vi "PSU_Keysight_34951A_SoftFP.vi"(0 "reference in":refnum<class "PSU_Keysight_34951A.lvclass">, 2 "Floating":bool, 5 "error in (no error)":errorcluster) -> (14 "reference out":refnum<class "PSU_Keysight_34951A.lvclass">, 19 "error out":errorcluster)   [LabVIEW 2022 SP3, in "PSU_Keysight_34951A.lvlib" / "PSU_Keysight_34951A.lvclass"]
uses:
  PSU_Keysight_34951A.lvclass
  Components/ViPER.lvlibp/ViPER.lvclass
  C:/Projects/Medulla/ViPER/Examples/Flux_Capacitor_Tester/Components/ViPER.lvlibp/ViPER.lvclass
panel:
  in  "C 4":T1 {"Current (A)" min=-0.02 max=0.02 step=0.001; "Voltage (V)" min=-16.0 max=16.0 step=0.01}
  in  "C 3":T1 {"Current (A)" min=-0.02 max=0.02 step=0.001; "Voltage (V)" min=-16.0 max=16.0 step=0.01}
  in  "C 2":T1 {"Current (A)" min=-0.02 max=0.02 step=0.001; "Voltage (V)" min=-16.0 max=16.0 step=0.01}
  in  "C1":T1 {"Current (A)" min=-0.02 max=0.02 step=0.001; "Voltage (V)" min=-16.0 max=16.0 step=0.01}
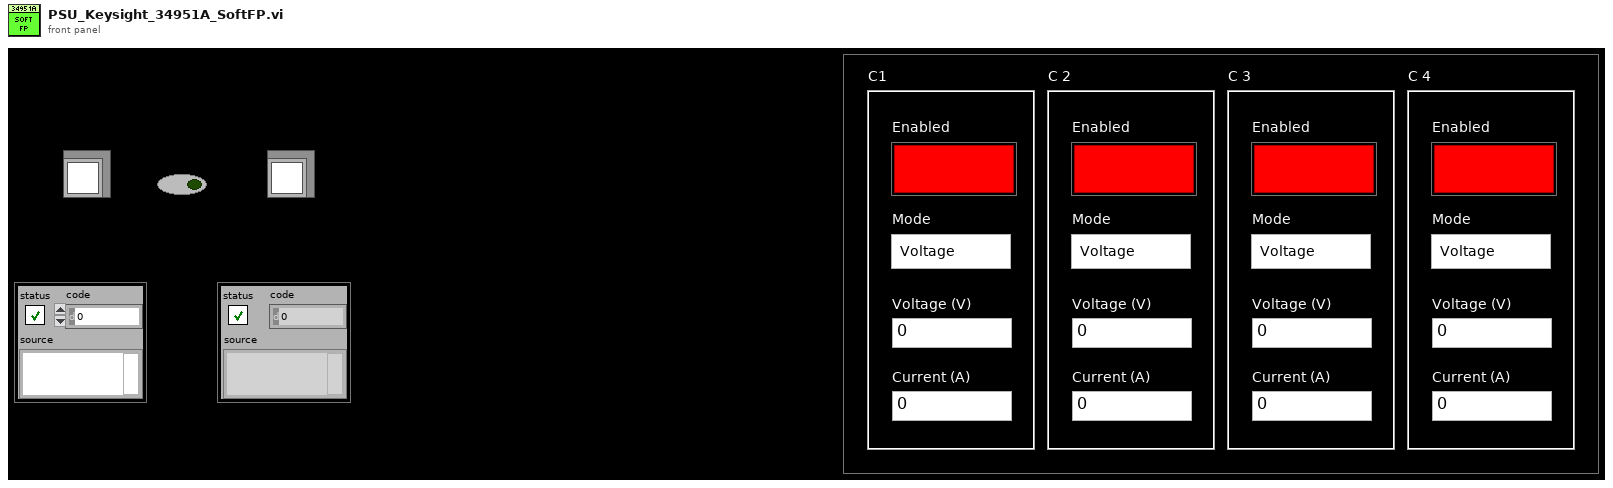
[diagram p1: front panel]
types:
  T1 = cluster{"Enabled":bool, "Mode":enum16{"Voltage", "Current"}, "Voltage (V)":dbl, "Current (A)":dbl}
  T2 = enum32{"Invalid", "Standard", "Closed", "Hidden", "Minimized", "Maximized"}
  T3 = typedef "PSU_Keysight_34951A.lvlib/PSU_Keysight_34951A.lvclass/ObjectAttributes.ctl" = cluster{"Config":T4, "VISA res":refnum<visa-resource-name>, "Enabled":bool[], "V":dbl[], "I":dbl[], "Source Type":enum16{"Voltage", "Current"}[]}
  T4 = typedef "PSU_Keysight_34951A.lvlib/PSU_Keysight_34951A.lvclass/Config.ctl" = cluster{"VISA":refnum<visa-resource-name>, "Slot":i32}
  T5 = cluster{"Enabled":bool, "Mode":bool, "Voltage (V)":bool, "Current (A)":bool}
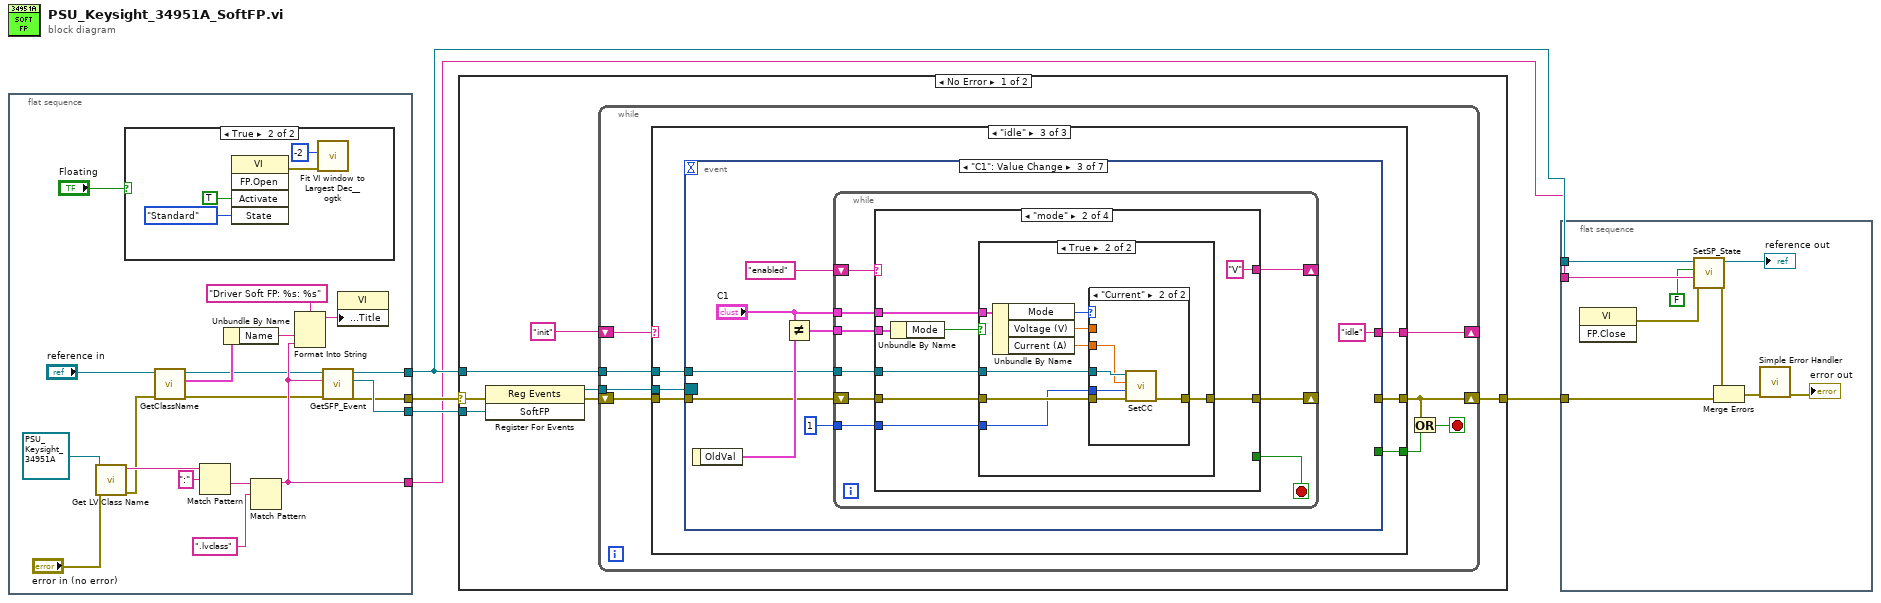
[diagram p0: block diagram]
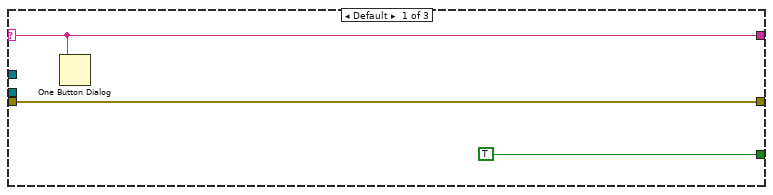
[diagram p3: hidden frame]
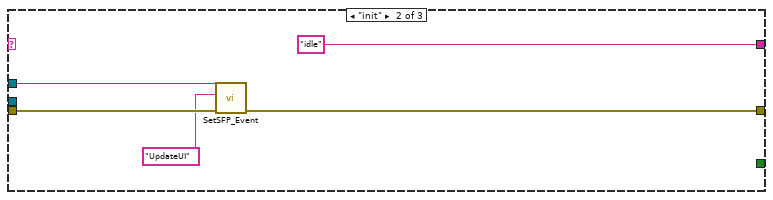
[diagram p4: hidden frame]
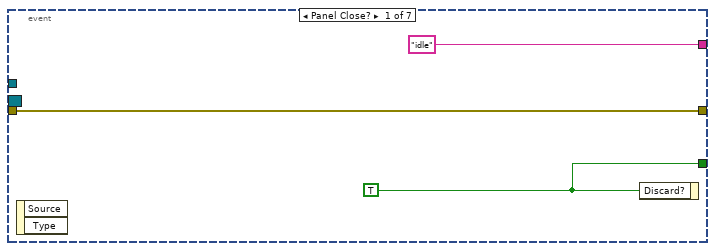
[diagram p5: hidden frame]
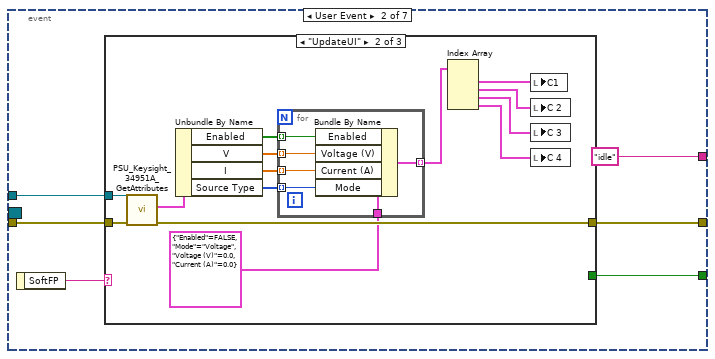
[diagram p6: hidden frame]
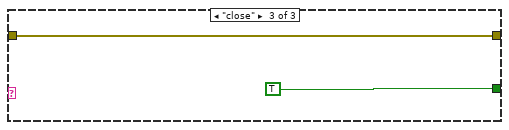
[diagram p8: hidden frame]
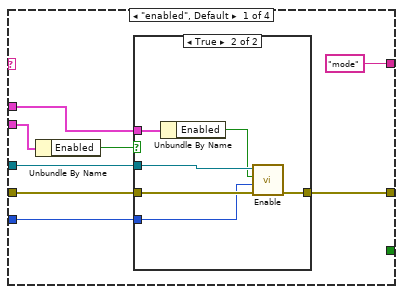
[diagram p9: hidden frame]
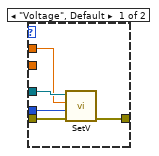
[diagram p12: hidden frame]
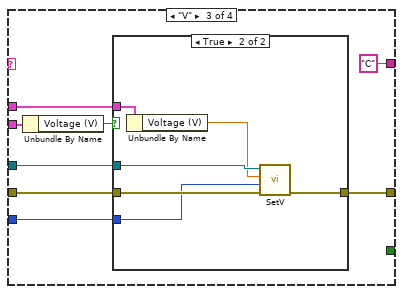
[diagram p13: hidden frame]
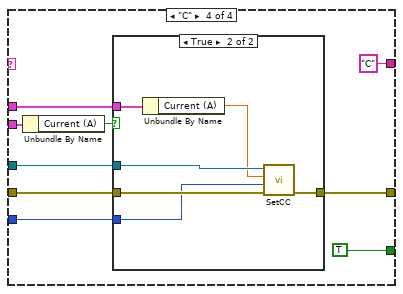
[diagram p15: hidden frame]
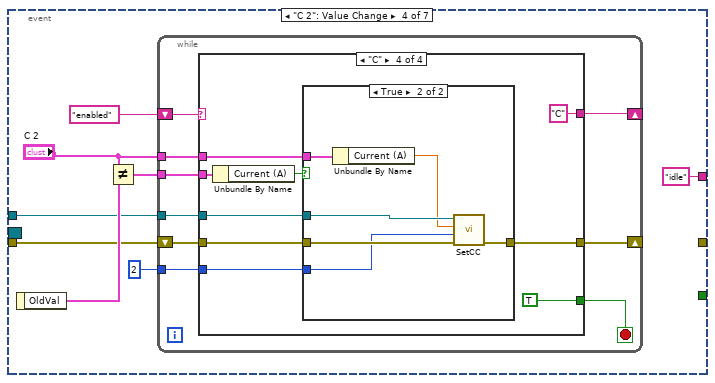
[diagram p17: hidden frame]
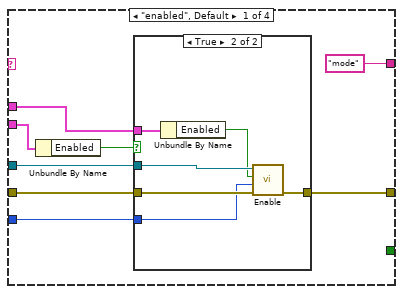
[diagram p18: hidden frame]
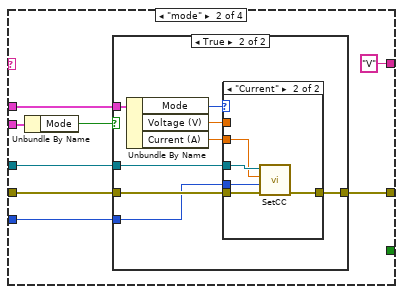
[diagram p20: hidden frame]
diagram:
  n1 = flat-sequence {
    tunnel: [w21] -> w5
    tunnel: [w20] -> w2
    tunnel: [w24] -> w3
    tunnel: [w12] -> w1
    frame #0 {
      n2 = call <vilib>:"Get LV Class Name.vi"("error in (no error)"="error in (no error)", "object"=refnum<class "PSU_Keysight_34951A.lvclass"> refnum ("reference")) -> ("error out"=w11:errorcluster, "class name"=w17:string)  [unwired: 8 in]
      n3 = case shown="True" "Floating" {
        frame False {
        }
        frame True {
          n4 = invoke class="VI" method="FP.Open"("Activate"=TRUE ("Activate?"), "State"=T2."Standard") -> (error out=w25:errorcluster)  [unwired: 3 in, 4 out]
          n5 = call <userlib>:"Fit VI window to Largest Dec__ogtk.vi"("error in (no error)"=w25, "border spacing (2 px)"=-2) -> ()  [unwired: 4 in, 2 out]
        }
      }
      n6 = call "GetClassName.vi"("error in (no error)"=w11, "reference in"="reference in") -> ("error out"=w10:errorcluster, "Details"=w9:cluster{"Name":string, "Class":string}, "reference out"=w7:refnum<class "PSU_Keysight_34951A.lvclass">)  [unwired: 7 in]
      n7 = Match Pattern(string=w17, regular expression=":") -> (after substring=w15:string)  [unwired: 1 in, 3 out]
      n8 = Unbundle By Name(w9) -> ("Name"=w19:string)
      n9 = Match Pattern(string=w15, regular expression=".lvclass") -> (before substring=w12:string)  [unwired: 1 in, 3 out]
      n10 = Format Into String(format string="Driver Soft FP: %s: %s", w19, w12) -> (resulting string=w23:string)  [unwired: 2 in, 1 out]
      n11 = call-dynamic "GetSFP_Event.vi"("error in (no error)"=w10, "Ancestor"=w12, "reference in"=w7) -> ("error out"=w21:errorcluster, "SoftFP"=w24:refnum<user-event>, "reference out"=w20:refnum<class "PSU_Keysight_34951A.lvclass">)  [unwired: 6 in]
      n12 = property class="VI"("Front Panel.Title"=w23) -> ()  [unwired: 2 in, 2 out]
    }
  }
  n13 = case shown="No Error" w5 {
    selector: w5 -> [w33 w452]
    tunnel: [w29 w452] -> w4
    tunnel: w2 -> [w30 _]
    tunnel: w3 -> [w35 _]
    frame No Error {
      n14 = register-events(error in=w33, w35) -> (reference out=w34:refnum<event-registration>, error out=w32:errorcluster)  [unwired: 1 in]
      n15 = while {
        shift-right: [w40] -> w29
        shift-left: w32 -> [w43]
        tunnel: w34 -> [w42]
        tunnel: w30 -> [w41]
        shift-right: [w36] -> _
        shift-left: "init" -> [w37]
        stop <- w39 stop-if-true
        n16 = case shown="\"idle\"" w37 {
          selector: w37 -> [w44 _ _]
          tunnel: w43 -> [w45 w49 w57]
          tunnel: w42 -> [_ _ w56]
          tunnel: w41 -> [_ w48 w55]
          tunnel: [w45 w50 w54] -> w40
          tunnel: [TRUE ("Discard?") _ w53] -> w38
          tunnel: [w44 "idle" w52] -> w36
          frame Default {
            n17 = One Button Dialog(message=w44) -> ()  [unwired: 1 in, 1 out]
          }
          frame "init" {
            n18 = call-dynamic "SetSFP_Event.vi"("error in (no error)"=w49, "msg"="UpdateUI" ("Ancestor"), "reference in"=w48) -> ("error out"=w50:errorcluster)  [unwired: 7 in, 1 out]
          }
          frame "idle" {
            n19 = event shown="[2] \"C1\": Value Change" {
              selector: w56 -> [_ _ _ _ _ _ _]
              dyn-events: _ -> [_ _ _ _ _ _ _]
              timeout: _ -> [_ _ _ _ _ _ _]
              tunnel: w57 -> [w60 w66 w91 w182 w272 w362 w451]
              tunnel: [w60 w64 _ _ _ _ w451] -> w54
              tunnel: [w59 w63 _ _ _ _ _] -> w53
              tunnel: w55 -> [_ w61 w90 w181 w271 w361 _]
              tunnel: ["idle" "idle" "idle" "idle" "idle" "idle" "idle"] -> w52
              event Panel Close? {
                w59 = TRUE ("Discard?")
                n20 = event-data() -> ()  [unwired: 1 in, 2 out]
                n21 = event-data("Discard?"=w59) -> ()  [unwired: 1 in, 1 out]
              }
              event User Event {
                n22 = event-data() -> ("SoftFP"=w65:string)  [unwired: 1 in]
                n23 = case shown="\"UpdateUI\"" w65 {
                  tunnel: w66 -> [w67 w81 w89]
                  tunnel: [w67 w79 w89] -> w64
                  tunnel: [_ _ TRUE ("Discard?")] -> w63
                  tunnel: w61 -> [_ w80 _]
                  frame Default {
                  }
                  frame "UpdateUI" {
                    n24 = call "PSU_Keysight_34951A_GetAttributes.vi"("error in (no error)"=w81, "reference in"=w80) -> ("error out"=w79:errorcluster, "Data"=w78:T3)  [unwired: 6 in, 2 out]
                    n25 = Unbundle By Name(w78) -> ("Enabled"=w77:bool[], "V"=w76:dbl[], "I"=w75:dbl[], "Source Type"=w74:enum16{"Voltage", "Current"}[])
                    n26 = for {
                      tunnel: w77 -> [w86] mode=indexing
                      tunnel: w76 -> [w85] mode=indexing
                      tunnel: w75 -> [w84] mode=indexing
                      tunnel: w74 -> [w83] mode=indexing
                      tunnel: T1 {"Enabled"=FALSE, "Mode"=enum."Voltage", "Voltage (V)"=0.0, "Current (A)"=0.0} ("C1") -> [w87]
                      tunnel: [w82] -> w72 mode=indexing
                      n27 = Bundle By Name(cluster=w87, "Enabled"=w86, "Voltage (V)"=w85, "Current (A)"=w84, "Mode"=w83) -> (w82:T1)
                    }
                    n28 = Index Array(array=w72) -> (element #1=w71:T1, element #2=w70:T1, element #3=w69:T1, element #4=w68:T1)  [unwired: 4 in]
                    n29 = local write "C1"(w71) -> ()
                    n30 = local write "C 2"(w70) -> ()
                    n31 = local write "C 3"(w69) -> ()
                    n32 = local write "C 4"(w68) -> ()
                  }
                  frame "close" {
                  }
                }
              }
              event "C1": Value Change {
                n33 = event-data() -> ("OldVal"=w97:T1)  [unwired: 1 in]
                n34 = Not Equal?(x="C1", y=w97) -> (x != y?=w95:T5)
                n35 = while {
                  tunnel: w95 -> [w105]
                  shift-right: [w98] -> _
                  shift-left: "enabled" -> [w106]
                  tunnel: "C1" -> [w104]
                  tunnel: 1 -> [w103]
                  shift-right: [w100] -> _
                  shift-left: w91 -> [w102]
                  tunnel: w90 -> [w101]
                  stop <- w99 stop-if-true
                  n36 = case shown="\"mode\"" w106 {
                    tunnel: w105 -> [w114 w129 w156 w172]
                    tunnel: w104 -> [w112 w127 w154 w170]
                    tunnel: w103 -> [w109 w124 w151 w167]
                    tunnel: w102 -> [w111 w126 w153 w169]
                    tunnel: w101 -> [w110 w125 w152 w168]
                    tunnel: [w108 w123 w150 w166] -> w100
                    tunnel: [_ _ _ TRUE] -> w99
                    tunnel: ["mode" "V" "C" "C"] -> w98
                    frame "enabled", Default {
                      n37 = Unbundle By Name(w114) -> ("Enabled"=w113:bool)
                      n38 = case shown="True" w113 {
                        tunnel: w112 -> [_ w121]
                        tunnel: w111 -> [w115 w119]
                        tunnel: w110 -> [_ w120]
                        tunnel: w109 -> [_ w117]
                        tunnel: [w115 w116] -> w108
                        frame False {
                        }
                        frame True {
                          n39 = Unbundle By Name(w121) -> ("Enabled"=w118:bool)
                          n40 = call-dynamic "Enable.vi"("error in (no error)"=w119, "Chan"=w117, "Enable"=w118, "reference in"=w120) -> ("error out"=w116:errorcluster)  [unwired: 6 in, 1 out]
                        }
                      }
                    }
                    frame "mode" {
                      n41 = Unbundle By Name(w129) -> ("Mode"=w128:bool)
                      n42 = case shown="True" w128 {
                        tunnel: w127 -> [_ w138]
                        tunnel: w126 -> [w130 w136]
                        tunnel: w125 -> [_ w137]
                        tunnel: w124 -> [_ w135]
                        tunnel: [w130 w134] -> w123
                        frame False {
                        }
                        frame True {
                          n43 = Unbundle By Name(w138) -> ("Mode"=w133:enum16{"Voltage", "Current"}, "Voltage (V)"=w132:dbl, "Current (A)"=w131:dbl)
                          n44 = case shown="\"Current\"" w133 {
                            tunnel: w137 -> [w141 w146]
                            tunnel: w136 -> [w143 w148]
                            tunnel: w135 -> [w140 w144]
                            tunnel: [w142 w147] -> w134
                            tunnel: w132 -> [w139 _]
                            tunnel: w131 -> [_ w145]
                            frame "Voltage", Default {
                              n45 = call-dynamic "SetV.vi"("error in (no error)"=w143, "Chan"=w140, "V"=w139, "reference in"=w141) -> ("error out"=w142:errorcluster)  [unwired: 6 in, 1 out]
                            }
                            frame "Current" {
                              n46 = call-dynamic "SetCC.vi"("error in (no error)"=w148, "Chan"=w144, "CC"=w145, "reference in"=w146) -> ("error out"=w147:errorcluster)  [unwired: 6 in, 1 out]
                            }
                          }
                        }
                      }
                    }
                    frame "V" {
                      n47 = Unbundle By Name(w156) -> ("Voltage (V)"=w155:bool)
                      n48 = case shown="True" w155 {
                        tunnel: w154 -> [_ w163]
                        tunnel: w153 -> [w157 w161]
                        tunnel: w152 -> [_ w162]
                        tunnel: w151 -> [_ w160]
                        tunnel: [w157 w159] -> w150
                        frame False {
                        }
                        frame True {
                          n49 = Unbundle By Name(w163) -> ("Voltage (V)"=w158:dbl)
                          n50 = call-dynamic "SetV.vi"("error in (no error)"=w161, "Chan"=w160, "V"=w158, "reference in"=w162) -> ("error out"=w159:errorcluster)  [unwired: 6 in, 1 out]
                        }
                      }
                    }
                    frame "C" {
                      n51 = Unbundle By Name(w172) -> ("Current (A)"=w171:bool)
                      n52 = case shown="True" w171 {
                        tunnel: w170 -> [_ w179]
                        tunnel: w169 -> [w173 w178]
                        tunnel: w168 -> [_ w176]
                        tunnel: w167 -> [_ w174]
                        tunnel: [w173 w177] -> w166
                        frame False {
                        }
                        frame True {
                          n53 = Unbundle By Name(w179) -> ("Current (A)"=w175:dbl)
                          n54 = call-dynamic "SetCC.vi"("error in (no error)"=w178, "Chan"=w174, "CC"=w175, "reference in"=w176) -> ("error out"=w177:errorcluster)  [unwired: 6 in, 1 out]
                        }
                      }
                    }
                  }
                }
              }
              event "C 2": Value Change {
                n55 = event-data() -> ("OldVal"=w187:T1)  [unwired: 1 in]
                n56 = Not Equal?(x="C 2", y=w187) -> (x != y?=w185:T5)
                n57 = while {
                  tunnel: w185 -> [w195]
                  shift-right: [w188] -> _
                  shift-left: "enabled" -> [w196]
                  tunnel: "C 2" -> [w194]
                  tunnel: 2 -> [w193]
                  shift-right: [w190] -> _
                  shift-left: w182 -> [w192]
                  tunnel: w181 -> [w191]
                  stop <- w189 stop-if-true
                  n58 = case shown="\"C\"" w196 {
                    tunnel: w195 -> [w204 w219 w246 w262]
                    tunnel: w194 -> [w202 w217 w244 w260]
                    tunnel: w193 -> [w199 w214 w241 w257]
                    tunnel: w192 -> [w201 w216 w243 w259]
                    tunnel: w191 -> [w200 w215 w242 w258]
                    tunnel: [w198 w213 w240 w256] -> w190
                    tunnel: [_ _ _ TRUE] -> w189
                    tunnel: ["mode" "V" "C" "C"] -> w188
                    frame "enabled", Default {
                      n59 = Unbundle By Name(w204) -> ("Enabled"=w203:bool)
                      n60 = case shown="True" w203 {
                        tunnel: w202 -> [_ w211]
                        tunnel: w201 -> [w205 w209]
                        tunnel: w200 -> [_ w210]
                        tunnel: w199 -> [_ w207]
                        tunnel: [w205 w206] -> w198
                        frame False {
                        }
                        frame True {
                          n61 = Unbundle By Name(w211) -> ("Enabled"=w208:bool)
                          n62 = call-dynamic "Enable.vi"("error in (no error)"=w209, "Chan"=w207, "Enable"=w208, "reference in"=w210) -> ("error out"=w206:errorcluster)  [unwired: 6 in, 1 out]
                        }
                      }
                    }
                    frame "mode" {
                      n63 = Unbundle By Name(w219) -> ("Mode"=w218:bool)
                      n64 = case shown="True" w218 {
                        tunnel: w217 -> [_ w228]
                        tunnel: w216 -> [w220 w226]
                        tunnel: w215 -> [_ w227]
                        tunnel: w214 -> [_ w225]
                        tunnel: [w220 w224] -> w213
                        frame False {
                        }
                        frame True {
                          n65 = Unbundle By Name(w228) -> ("Mode"=w223:enum16{"Voltage", "Current"}, "Voltage (V)"=w222:dbl, "Current (A)"=w221:dbl)
                          n66 = case shown="\"Current\"" w223 {
                            tunnel: w227 -> [w231 w236]
                            tunnel: w226 -> [w233 w238]
                            tunnel: w225 -> [w230 w234]
                            tunnel: [w232 w237] -> w224
                            tunnel: w222 -> [w229 _]
                            tunnel: w221 -> [_ w235]
                            frame "Voltage", Default {
                              n67 = call-dynamic "SetV.vi"("error in (no error)"=w233, "Chan"=w230, "V"=w229, "reference in"=w231) -> ("error out"=w232:errorcluster)  [unwired: 6 in, 1 out]
                            }
                            frame "Current" {
                              n68 = call-dynamic "SetCC.vi"("error in (no error)"=w238, "Chan"=w234, "CC"=w235, "reference in"=w236) -> ("error out"=w237:errorcluster)  [unwired: 6 in, 1 out]
                            }
                          }
                        }
                      }
                    }
                    frame "V" {
                      n69 = Unbundle By Name(w246) -> ("Voltage (V)"=w245:bool)
                      n70 = case shown="True" w245 {
                        tunnel: w244 -> [_ w253]
                        tunnel: w243 -> [w247 w251]
                        tunnel: w242 -> [_ w252]
                        tunnel: w241 -> [_ w250]
                        tunnel: [w247 w249] -> w240
                        frame False {
                        }
                        frame True {
                          n71 = Unbundle By Name(w253) -> ("Voltage (V)"=w248:dbl)
                          n72 = call-dynamic "SetV.vi"("error in (no error)"=w251, "Chan"=w250, "V"=w248, "reference in"=w252) -> ("error out"=w249:errorcluster)  [unwired: 6 in, 1 out]
                        }
                      }
                    }
                    frame "C" {
                      n73 = Unbundle By Name(w262) -> ("Current (A)"=w261:bool)
                      n74 = case shown="True" w261 {
                        tunnel: w260 -> [_ w269]
                        tunnel: w259 -> [w263 w268]
                        tunnel: w258 -> [_ w266]
                        tunnel: w257 -> [_ w264]
                        tunnel: [w263 w267] -> w256
                        frame False {
                        }
                        frame True {
                          n75 = Unbundle By Name(w269) -> ("Current (A)"=w265:dbl)
                          n76 = call-dynamic "SetCC.vi"("error in (no error)"=w268, "Chan"=w264, "CC"=w265, "reference in"=w266) -> ("error out"=w267:errorcluster)  [unwired: 6 in, 1 out]
                        }
                      }
                    }
                  }
                }
              }
              event "C 3": Value Change {
                n77 = event-data() -> ("OldVal"=w277:T1)  [unwired: 1 in]
                n78 = Not Equal?(x="C 3", y=w277) -> (x != y?=w275:T5)
                n79 = while {
                  tunnel: w275 -> [w285]
                  shift-right: [w278] -> _
                  shift-left: "enabled" -> [w286]
                  tunnel: "C 3" -> [w284]
                  tunnel: 3 -> [w283]
                  shift-right: [w280] -> _
                  shift-left: w272 -> [w282]
                  tunnel: w271 -> [w281]
                  stop <- w279 stop-if-true
                  n80 = case shown="\"C\"" w286 {
                    tunnel: w285 -> [w294 w309 w336 w352]
                    tunnel: w284 -> [w292 w307 w334 w350]
                    tunnel: w283 -> [w289 w304 w331 w347]
                    tunnel: w282 -> [w291 w306 w333 w349]
                    tunnel: w281 -> [w290 w305 w332 w348]
                    tunnel: [w288 w303 w330 w346] -> w280
                    tunnel: [_ _ _ TRUE] -> w279
                    tunnel: ["mode" "V" "C" "C"] -> w278
                    frame "enabled", Default {
                      n81 = Unbundle By Name(w294) -> ("Enabled"=w293:bool)
                      n82 = case shown="True" w293 {
                        tunnel: w292 -> [_ w301]
                        tunnel: w291 -> [w295 w299]
                        tunnel: w290 -> [_ w300]
                        tunnel: w289 -> [_ w297]
                        tunnel: [w295 w296] -> w288
                        frame False {
                        }
                        frame True {
                          n83 = Unbundle By Name(w301) -> ("Enabled"=w298:bool)
                          n84 = call-dynamic "Enable.vi"("error in (no error)"=w299, "Chan"=w297, "Enable"=w298, "reference in"=w300) -> ("error out"=w296:errorcluster)  [unwired: 6 in, 1 out]
                        }
                      }
                    }
                    frame "mode" {
                      n85 = Unbundle By Name(w309) -> ("Mode"=w308:bool)
                      n86 = case shown="True" w308 {
                        tunnel: w307 -> [_ w318]
                        tunnel: w306 -> [w310 w316]
                        tunnel: w305 -> [_ w317]
                        tunnel: w304 -> [_ w315]
                        tunnel: [w310 w314] -> w303
                        frame False {
                        }
                        frame True {
                          n87 = Unbundle By Name(w318) -> ("Mode"=w313:enum16{"Voltage", "Current"}, "Voltage (V)"=w312:dbl, "Current (A)"=w311:dbl)
                          n88 = case shown="\"Current\"" w313 {
                            tunnel: w317 -> [w321 w326]
                            tunnel: w316 -> [w323 w328]
                            tunnel: w315 -> [w320 w324]
                            tunnel: [w322 w327] -> w314
                            tunnel: w312 -> [w319 _]
                            tunnel: w311 -> [_ w325]
                            frame "Voltage", Default {
                              n89 = call-dynamic "SetV.vi"("error in (no error)"=w323, "Chan"=w320, "V"=w319, "reference in"=w321) -> ("error out"=w322:errorcluster)  [unwired: 6 in, 1 out]
                            }
                            frame "Current" {
                              n90 = call-dynamic "SetCC.vi"("error in (no error)"=w328, "Chan"=w324, "CC"=w325, "reference in"=w326) -> ("error out"=w327:errorcluster)  [unwired: 6 in, 1 out]
                            }
                          }
                        }
                      }
                    }
                    frame "V" {
                      n91 = Unbundle By Name(w336) -> ("Voltage (V)"=w335:bool)
                      n92 = case shown="True" w335 {
                        tunnel: w334 -> [_ w343]
                        tunnel: w333 -> [w337 w341]
                        tunnel: w332 -> [_ w342]
                        tunnel: w331 -> [_ w340]
                        tunnel: [w337 w339] -> w330
                        frame False {
                        }
                        frame True {
                          n93 = Unbundle By Name(w343) -> ("Voltage (V)"=w338:dbl)
                          n94 = call-dynamic "SetV.vi"("error in (no error)"=w341, "Chan"=w340, "V"=w338, "reference in"=w342) -> ("error out"=w339:errorcluster)  [unwired: 6 in, 1 out]
                        }
                      }
                    }
                    frame "C" {
                      n95 = Unbundle By Name(w352) -> ("Current (A)"=w351:bool)
                      n96 = case shown="True" w351 {
                        tunnel: w350 -> [_ w359]
                        tunnel: w349 -> [w353 w358]
                        tunnel: w348 -> [_ w356]
                        tunnel: w347 -> [_ w354]
                        tunnel: [w353 w357] -> w346
                        frame False {
                        }
                        frame True {
                          n97 = Unbundle By Name(w359) -> ("Current (A)"=w355:dbl)
                          n98 = call-dynamic "SetCC.vi"("error in (no error)"=w358, "Chan"=w354, "CC"=w355, "reference in"=w356) -> ("error out"=w357:errorcluster)  [unwired: 6 in, 1 out]
                        }
                      }
                    }
                  }
                }
              }
              event "C 4": Value Change {
                n99 = event-data() -> ("OldVal"=w367:T1)  [unwired: 1 in]
                n100 = Not Equal?(x="C 4", y=w367) -> (x != y?=w365:T5)
                n101 = while {
                  tunnel: w365 -> [w375]
                  shift-right: [w368] -> _
                  shift-left: "enabled" -> [w376]
                  tunnel: "C 4" -> [w374]
                  tunnel: 4 -> [w373]
                  shift-right: [w370] -> _
                  shift-left: w362 -> [w372]
                  tunnel: w361 -> [w371]
                  stop <- w369 stop-if-true
                  n102 = case shown="\"C\"" w376 {
                    tunnel: w375 -> [w384 w399 w426 w442]
                    tunnel: w374 -> [w382 w397 w424 w440]
                    tunnel: w373 -> [w379 w394 w421 w437]
                    tunnel: w372 -> [w381 w396 w423 w439]
                    tunnel: w371 -> [w380 w395 w422 w438]
                    tunnel: [w378 w393 w420 w436] -> w370
                    tunnel: [_ _ _ TRUE] -> w369
                    tunnel: ["mode" "V" "C" "C"] -> w368
                    frame "enabled", Default {
                      n103 = Unbundle By Name(w384) -> ("Enabled"=w383:bool)
                      n104 = case shown="True" w383 {
                        tunnel: w382 -> [_ w391]
                        tunnel: w381 -> [w385 w389]
                        tunnel: w380 -> [_ w390]
                        tunnel: w379 -> [_ w387]
                        tunnel: [w385 w386] -> w378
                        frame False {
                        }
                        frame True {
                          n105 = Unbundle By Name(w391) -> ("Enabled"=w388:bool)
                          n106 = call-dynamic "Enable.vi"("error in (no error)"=w389, "Chan"=w387, "Enable"=w388, "reference in"=w390) -> ("error out"=w386:errorcluster)  [unwired: 6 in, 1 out]
                        }
                      }
                    }
                    frame "mode" {
                      n107 = Unbundle By Name(w399) -> ("Mode"=w398:bool)
                      n108 = case shown="True" w398 {
                        tunnel: w397 -> [_ w408]
                        tunnel: w396 -> [w400 w406]
                        tunnel: w395 -> [_ w407]
                        tunnel: w394 -> [_ w405]
                        tunnel: [w400 w404] -> w393
                        frame False {
                        }
                        frame True {
                          n109 = Unbundle By Name(w408) -> ("Mode"=w403:enum16{"Voltage", "Current"}, "Voltage (V)"=w402:dbl, "Current (A)"=w401:dbl)
                          n110 = case shown="\"Current\"" w403 {
                            tunnel: w407 -> [w411 w416]
                            tunnel: w406 -> [w413 w418]
                            tunnel: w405 -> [w410 w414]
                            tunnel: [w412 w417] -> w404
                            tunnel: w402 -> [w409 _]
                            tunnel: w401 -> [_ w415]
                            frame "Voltage", Default {
                              n111 = call-dynamic "SetV.vi"("error in (no error)"=w413, "Chan"=w410, "V"=w409, "reference in"=w411) -> ("error out"=w412:errorcluster)  [unwired: 6 in, 1 out]
                            }
                            frame "Current" {
                              n112 = call-dynamic "SetCC.vi"("error in (no error)"=w418, "Chan"=w414, "CC"=w415, "reference in"=w416) -> ("error out"=w417:errorcluster)  [unwired: 6 in, 1 out]
                            }
                          }
                        }
                      }
                    }
                    frame "V" {
                      n113 = Unbundle By Name(w426) -> ("Voltage (V)"=w425:bool)
                      n114 = case shown="True" w425 {
                        tunnel: w424 -> [_ w433]
                        tunnel: w423 -> [w427 w431]
                        tunnel: w422 -> [_ w432]
                        tunnel: w421 -> [_ w430]
                        tunnel: [w427 w429] -> w420
                        frame False {
                        }
                        frame True {
                          n115 = Unbundle By Name(w433) -> ("Voltage (V)"=w428:dbl)
                          n116 = call-dynamic "SetV.vi"("error in (no error)"=w431, "Chan"=w430, "V"=w428, "reference in"=w432) -> ("error out"=w429:errorcluster)  [unwired: 6 in, 1 out]
                        }
                      }
                    }
                    frame "C" {
                      n117 = Unbundle By Name(w442) -> ("Current (A)"=w441:bool)
                      n118 = case shown="True" w441 {
                        tunnel: w440 -> [_ w449]
                        tunnel: w439 -> [w443 w448]
                        tunnel: w438 -> [_ w446]
                        tunnel: w437 -> [_ w444]
                        tunnel: [w443 w447] -> w436
                        frame False {
                        }
                        frame True {
                          n119 = Unbundle By Name(w449) -> ("Current (A)"=w445:dbl)
                          n120 = call-dynamic "SetCC.vi"("error in (no error)"=w448, "Chan"=w444, "CC"=w445, "reference in"=w446) -> ("error out"=w447:errorcluster)  [unwired: 6 in, 1 out]
                        }
                      }
                    }
                  }
                }
              }
              event Timeout {
                n121 = event-data() -> ()  [unwired: 1 in, 2 out]
              }
            }
          }
        }
        n122 = Or(x=w40, y=w38) -> (x .or. y?=w39:bool)
      }
    }
    frame Error {
    }
  }
  n123 = flat-sequence {
    tunnel: w4 -> [w459]
    tunnel: w2 -> [w454]
    tunnel: w1 -> [w456]
    frame #0 {
      n124 = invoke class="VI" method="FP.Close"() -> (error out=w458:errorcluster)  [unwired: 3 in, 2 out]
      n125 = call "SetSP_State.vi"("error in (no error)"=w458, "Ancestor"=w456, "SP Open"=FALSE, "reference in"=w454) -> ("error out"=w457:errorcluster, "reference out"=→"reference out":refnum<class "PSU_Keysight_34951A.lvclass">)  [unwired: 6 in]
      n126 = Merge Errors(w457, w459) -> (w461:errorcluster)
      n127 = call <vilib>:"Simple Error Handler.vi"("error in (no error)"=w461) -> ("error out"=→"error out":errorcluster)  [unwired: 4 in, 4 out]
    }
  }
